vi "Change deadband constants for a faster stop.vi"(10 "Quick stop":bool, 11 "Deadbands in":T1) -> (3 "Deadbands out":T1)   [LabVIEW 2013]
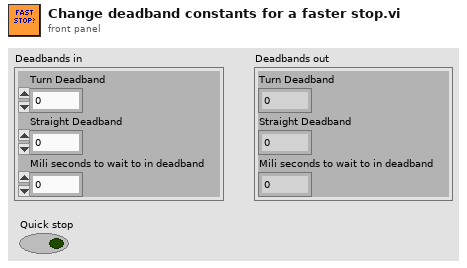
[diagram p1: front panel]
types:
  T1 = cluster{"Turn Deadband":dbl, "Straight Deadband":dbl, "Mili seconds to wait to in deadband":u32}
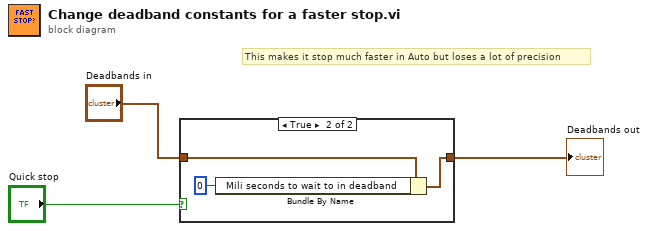
[diagram p0: block diagram]
diagram:
  # "This makes it stop much faster in Auto but loses a lot of precision"
  n1 = case shown="True" "Quick stop" {
    tunnel: "Deadbands in" -> [w4 w7]
    tunnel: [w4 w6] -> w2
    frame False {
    }
    frame True {
      n2 = Bundle By Name(cluster=w7, "Mili seconds to wait to in deadband"=u32 0) -> (w6:T1)
    }
  }
  "Deadbands out" <- w2
